vi "GetCurrent.vi"(4 "error in":errorcluster, 5 "connection ID":refnum<k5>) -> (0 "Current":string, 1 "error out":errorcluster, 2 "connection ID out":refnum<k5>, 3 "Answer":bool)   [LabVIEW 2013]
panel:
  out "читаю hex":string
  out "читаю текст":string
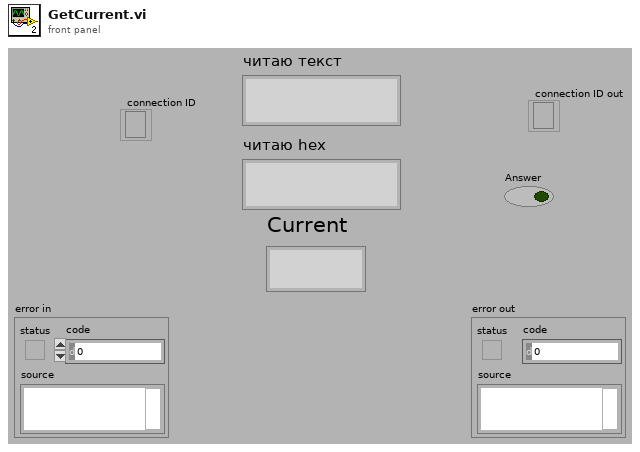
[diagram p1: front panel]
types:
  T1 = enum16{"Standard", "Buffered", "CRLF", "Immediate"}
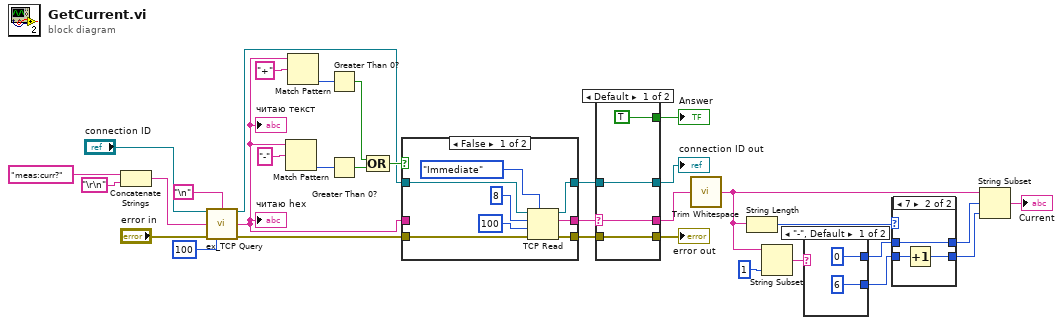
[diagram p0: block diagram]
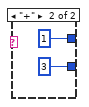
[diagram p3: hidden frame]
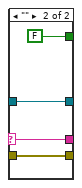
[diagram p5: hidden frame]
diagram:
  n1 = Concatenate Strings("meas:curr?" ("data in"), "\r\n") -> (w8:string)
  n2 = call "ex_TCP Query.vi"("TCP Network Connection in"="connection ID", "Termination character"="\n", "Query string"=w8, "error in (no error)"="error in", "Initial byte timeout ms (1000)"=100) -> ("TCP Network Connection out"=w4:refnum<k5>, "Message data out"=w2:string, "error out"=w3:errorcluster)  [unwired: 7 in, 1 out]
  "читаю hex" <- w2
  "читаю текст" <- w2
  n3 = Match Pattern(string=w2, regular expression="-") -> (offset past match=w22:i32)  [unwired: 1 in, 3 out]
  n4 = Match Pattern(string=w2, regular expression="+") -> (offset past match=w31:i32)  [unwired: 1 in, 3 out]
  n5 = Greater Than 0?(x=w31) -> (x > 0?=w21:bool)
  n6 = Greater Than 0?(x=w22) -> (x > 0?=w20:bool)
  n7 = Compound Arithmetic op=OR(w21, w20) -> (w19:bool)
  n8 = case shown="False" w19 {
    tunnel: w2 -> [_ w44]
    tunnel: [w34 w44] -> w26
    tunnel: w4 -> [w38 w43]
    tunnel: [w37 w43] -> w25
    tunnel: w3 -> [w36 w42]
    tunnel: [w35 w42] -> w24
    frame False {
      n9 = TCP Read(connection ID=w38, bytes to read=8, error in (no error)=w36, 7:T1."Immediate" ("mode (standard)"), 9:100 ("timeout ms (25000)")) -> (connection ID out=w37:refnum<k5>, data out=w34:string, error out=w35:errorcluster)
    }
    frame True {
    }
  }
  n10 = case shown="Default" w26 {
    selector: w26 -> [w48 w52]
    tunnel: [w48 w52] -> w17
    tunnel: [TRUE FALSE] -> w27
    tunnel: w24 -> [w46 w50]
    tunnel: [w46 w50] -> w29
    tunnel: w25 -> [w45 w49]
    tunnel: [w45 w49] -> w30
    frame Default {
    }
    frame "" {
    }
  }
  "Answer" <- w27
  "connection ID out" <- w30
  "error out" <- w29
  n11 = call <vilib>:"Trim Whitespace.vi"("string"=w17) -> ("trimmed string"=w14:string)  [unwired: 1 in]
  n12 = String Length(string=w14) -> (length=w13:i32)
  n13 = String Subset(string=w14, length (rest)=1 ("length (rest)")) -> (substring=w16:string)  [unwired: 1 in]
  n14 = case shown="\"-\", Default" w16 {
    tunnel: [0 ("length (rest)") 1 ("length (rest)")] -> w10
    tunnel: [6 ("length (rest)") 3 ("length (rest)")] -> w12
    frame "-", Default {
    }
    frame "+" {
    }
  }
  n15 = case shown="7" w13 {
    tunnel: w12 -> [w58 w61]
    tunnel: [w58 w60] -> w11
    tunnel: w10 -> [w57 w59]
    tunnel: [w57 w59] -> w9
    frame 6, Default {
    }
    frame 7 {
      n16 = Increment(x=w61) -> (x+1=w60:i32)
    }
  }
  n17 = String Subset(string=w14, offset (0)=w9, length (rest)=w11) -> (substring=→"Current":string)
